vi "SPARK Get Absolute Encoder Status.vi"   [LabVIEW 2023]
doc: "Get the periodic status from an absolute encoder connected to the data port of the SPARK."
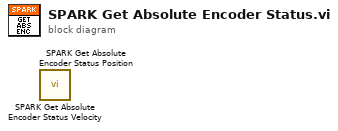
[diagram p0: block diagram]
diagram:
  n1 = call "SPARK Get Absolute Encoder Status Velocity.vi"() -> ()  [unwired: 8 in, 4 out]
  n2 = call "SPARK Get Absolute Encoder Status Position.vi"() -> ()  [unwired: 8 in, 4 out]
